vi "CTRE_CANifier_EnablePWMOutput.vi"(8 "error in":errorcluster, 9 "PWMChannel":T1, 10 "Enable?":bool=TRUE, 11 "CANifierDevRef":T2) -> (0 "error out":errorcluster, 3 "CANifierDevRef":T2)   [LabVIEW 2016]
uses:
  <vilib>/Rock Robotics/WPI/ThirdParty/Sensors/CANifier/CTRE_CANifier_DeviceRef.ctl
  <vilib>/Rock Robotics/WPI/ThirdParty/Sensors/CANifier/CTRE_CANifier_PWMChannel.ctl
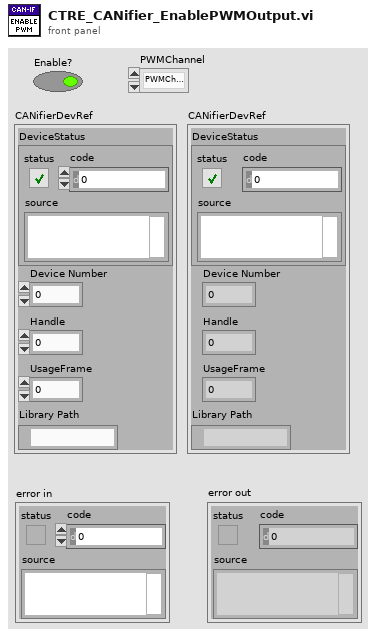
[diagram p1: front panel]
types:
  T1 = typedef "CTRE_CANifier_PWMChannel.ctl" = enum16{"PWMChannel0", "PWMChannel1", "PWMChannel2", "PWMChannel3"}
  T2 = typedef "CTRE_CANifier_DeviceRef.ctl" = cluster{"DeviceStatus":errorcluster, "Device Number":u8, "Handle":u64, "UsageFrame":u32, "Library Path":path}
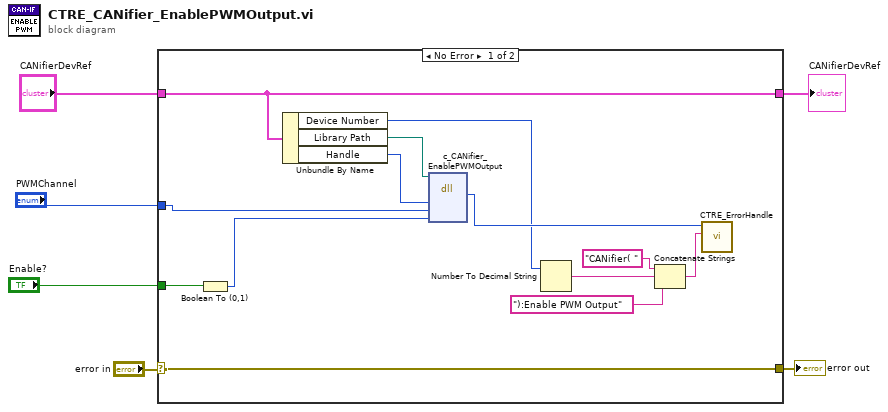
[diagram p0: block diagram]
diagram:
  n1 = case shown="No Error" "error in" {
    selector: "error in" -> [w19 w21]
    tunnel: [w19 w21] -> w5
    tunnel: "PWMChannel" -> [w9 _]
    tunnel: "CANifierDevRef" -> [w18 w20]
    tunnel: [w18 w20] -> w3
    tunnel: "Enable?" -> [w8 _]
    frame No Error {
      n2 = Boolean To (0,1)(Boolean=w8) -> (0, 1=w7:i16)
      n3 = Unbundle By Name(w18) -> ("Device Number"=w11:u8, "Library Path"=w17:path, "Handle"=w16:u64)
      n4 = dll-call lib="?" fn="c_CANifier_EnablePWMOutput"(path in=w17, "handle"=w16, "pwmChannel"=w9, "bEnable"=w7) -> ("CTR_Code"=w15:i8)  [unwired: 5 in, 2 out]
      n5 = Number To Decimal String(number=w11) -> (decimal integer string=w14:string)  [unwired: 1 in]
      n6 = Concatenate Strings("CANifier( " ("string"), w14, "):Enable PWM Output" ("string")) -> (w10:string)
      n7 = call <vilib>:"CTRE_ErrorHandle.vi"("origin"=w10, "code"=w15) -> ()  [unwired: 9 in, 1 out]
    }
    frame Error {
    }
  }
  "error out" <- w5
  "CANifierDevRef" <- w3
